vi "CSMP-PostSendMsg.vi"(0 "state":string, 1 "args":string, 2 "source/target":string, 5 "Error in":errorcluster caption="Error in (no error)", 6 "session error":errorcluster, 8 "Module Name":string, 10 "Response Arguments":string) -> (14 "state out":string, 15 "args out":string, 16 "source/target out":string, 19 "error":errorcluster)   [LabVIEW 2020, in "Communicable State Machine.lvlib"]
uses:
  Communicable State Machine.lvlib
  _Cross CSM State Response.ctl
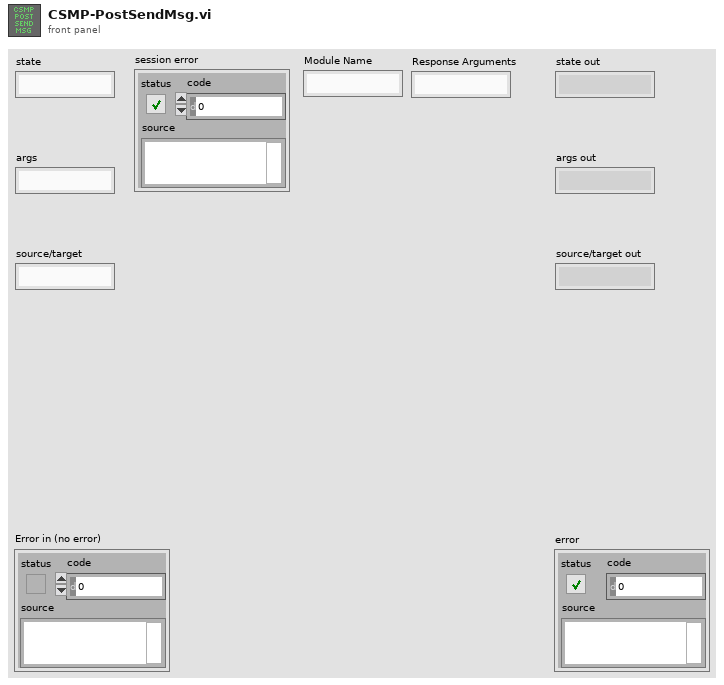
[diagram p1: front panel]
types:
  T1 = typedef "Communicable State Machine.lvlib/_Cross CSM State Response.ctl" = cluster{"error":errorcluster, "Response Data":string, "From Who":string}
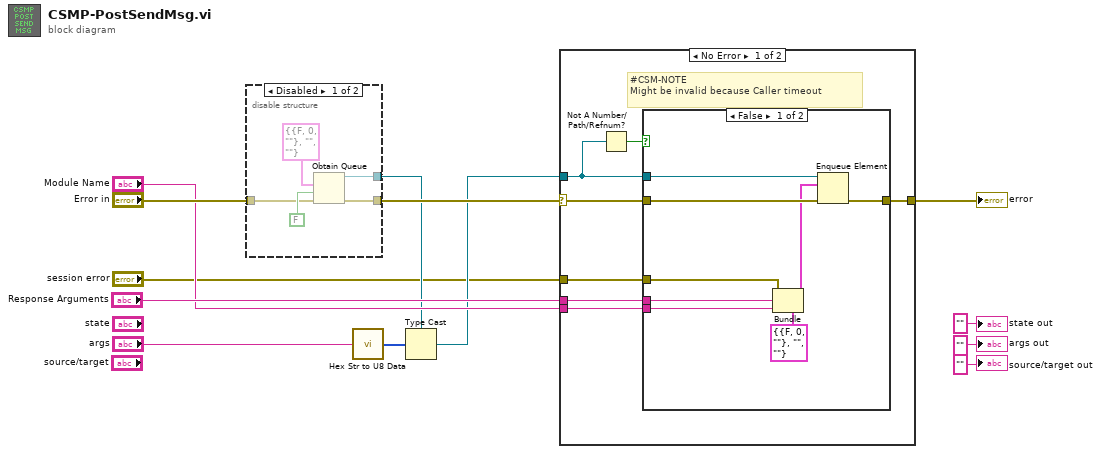
[diagram p0: block diagram]
diagram:
  n1 = disable-structure shown="Disabled" {
    disable-tunnel: [w18 _] -> w5
    disable-tunnel: [w17 _] -> w13
    disable-tunnel: "Error in" -> [w14 _]
    frame Disabled {
      n2 = Obtain Queue(element data type=T1 {"error"={"status"=FALSE, "code"=0, "source"=""}, "Response Data"="", "From Who"=""} ("Cross JKI State Machine Response"), create if not found? (T)=FALSE, error in (no error)=w14) -> (queue out=w18:refnum<queue>, error out=w17:errorcluster)  [unwired: 2 in, 1 out]
    }
    frame Enabled {
    }
  }
  n3 = call "Hex Str to U8 Data.vi"("HEX String (0-9,A-F)"="args") -> ("u8 Data[]"=w2:u8[])
  n4 = Type Cast(type=w5, x=w2) -> (*(type *) &x=w4:refnum<queue>)
  n5 = case shown="No Error" w13 {
    selector: w13 -> [w25 w35]
    tunnel: w4 -> [w21 _]
    tunnel: [w24 w35] -> w6
    tunnel: "Module Name" -> [w23 _]
    tunnel: "Response Arguments" -> [w22 _]
    tunnel: "session error" -> [w19 _]
    frame No Error {
      # "#CSM-NOTE\nMight be invalid because Caller timeout"
      n6 = Not A Number/Path/Refnum?(number/path/refnum=w21) -> (NaN/Path/Refnum?=w20:bool)
      n7 = case shown="False" w20 {
        tunnel: w25 -> [w33 w34]
        tunnel: [w32 w34] -> w24
        tunnel: w23 -> [w29 _]
        tunnel: w22 -> [w28 _]
        tunnel: w21 -> [w27 _]
        tunnel: w19 -> [w26 _]
        frame False {
          n8 = Bundle(cluster=T1 {"error"={"status"=FALSE, "code"=0, "source"=""}, "Response Data"="", "From Who"=""} ("element"), "error"=w26, "Response Data"=w28, "From Who"=w29) -> (w30:T1)
          n9 = Enqueue Element(queue=w27, element=w30, error in (no error)=w33) -> (error out=w32:errorcluster)  [unwired: 1 in, 2 out]
        }
        frame True {
        }
      }
    }
    frame Error {
    }
  }
  "error" <- w6
  "state out" <- "" ("Pre-State out")
  "args out" <- "" ("Pre-State out")
  "source/target out" <- "" ("Pre-Args out")
